vi "ConfigurePeeling.vi"(8 "error in (no error)":errorcluster, 11 "BananaPeel in":refnum<class "BananaPeel.lvclass">) -> (0 "error out":errorcluster, 3 "BananaPeel out":refnum<class "BananaPeel.lvclass">)   [LabVIEW 2021, in "Bananas.lvlib" / "BananaPeel.lvclass"]
uses:
  BananaPeel.lvclass
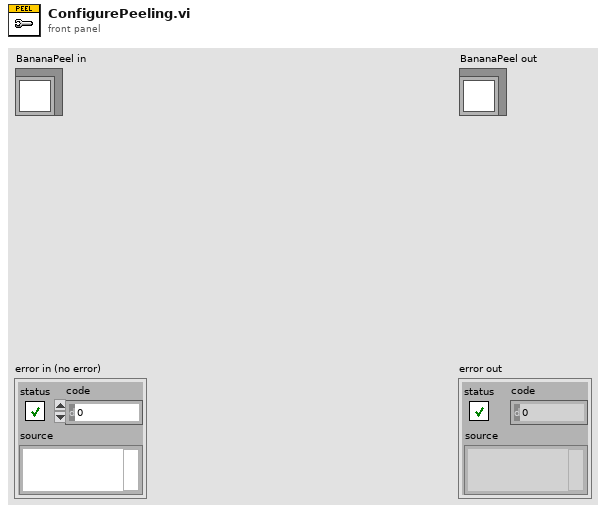
[diagram p1: front panel]
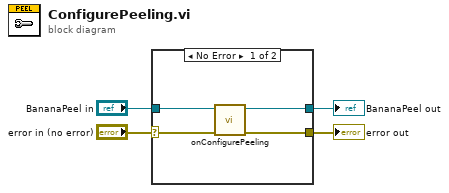
[diagram p0: block diagram]
diagram:
  n1 = case shown="No Error" "error in (no error)" {
    selector: "error in (no error)" -> [w6 w10]
    tunnel: [w5 w10] -> w3
    tunnel: [w8 w9] -> w1
    tunnel: "BananaPeel in" -> [w7 w9]
    frame No Error {
      n2 = call-dynamic "onConfigurePeeling.vi"("error in (no error)"=w6, "BananaPeel in"=w7) -> ("error out"=w5:errorcluster, "BananaPeel out"=w8:refnum<class "BananaPeel.lvclass">)  [unwired: 8 in]
    }
    frame Error {
    }
  }
  "error out" <- w3
  "BananaPeel out" <- w1
